vi "Main.vi"() -> ()   [LabVIEW 2020, in "BubbleSortvi.lvlib"]
uses:
  BubbleSortvi.lvlib
panel:
  out "SORTED ARRAY":dbl[](array[numeric])
  in  "UNSORTED ARRAY":dbl[](array[numeric])=[5.0, 15.0, 2.0, 1.0, 9.0, 20.0]
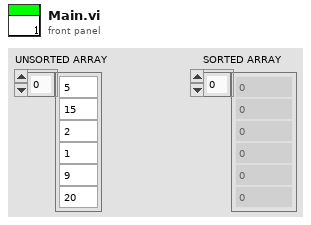
[diagram p1: front panel]
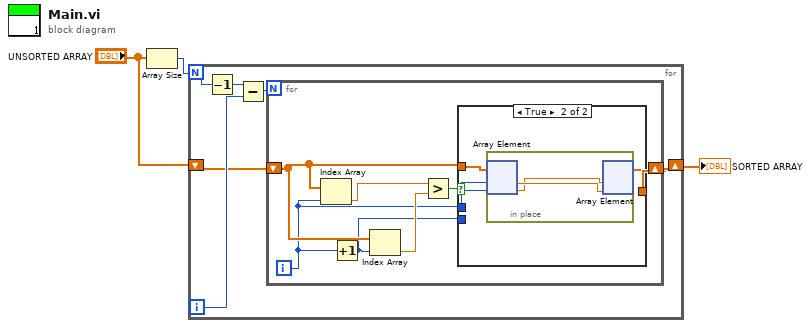
[diagram p0: block diagram]
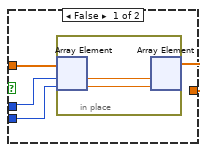
[diagram p2: hidden frame]
diagram:
  n1 = Array Size(array="UNSORTED ARRAY") -> (size(s)=w3:i32)
  n2 = for {
    N: w3 -> [w9]
    shift-right: [w4] -> w1
    shift-left: "UNSORTED ARRAY" -> [w5]
    i -> [w7]
    n3 = Decrement(x=w9) -> (x-1=w8:i32)
    n4 = Subtract(x=w8, y=w7) -> (x-y=w6:i32)
    n5 = for {
      N: w6 -> [_]
      shift-right: [w10] -> w4
      shift-left: w5 -> [w13]
      i -> [w12]
      n6 = Index Array(array=w13, index=w12) -> (element=w16:dbl)
      n7 = Increment(x=w12) -> (x+1=w11:i32)
      n8 = Index Array(array=w13, index=w11) -> (element=w15:dbl)
      n9 = Greater?(x=w16, y=w15) -> (0:w14:bool)
      n10 = case shown="True" w14 {
        tunnel: w13 -> [w20 w24]
        tunnel: w12 -> [w19 w26]
        tunnel: w11 -> [w18 w25]
        tunnel: [w17 w23] -> w10
        frame False {
          n11 = in-place {
            n12 = in-place-array #1(w20, w19, w18) -> (w22:dbl, w21:dbl)
            n13 = in-place-array #1(w22, w21) -> (w17:dbl[])  [unwired: 2 out]
          }
        }
        frame True {
          n14 = in-place {
            n15 = in-place-array #2(w24, w26, w25) -> (w28:dbl, w27:dbl)
            n16 = in-place-array #2(w27, w28) -> (w23:dbl[])  [unwired: 2 out]
          }
        }
      }
    }
  }
  "SORTED ARRAY" <- w1
